vi "Find Top Level.vi"(8 "error in (no error)":errorcluster, 10 "VI":string) -> (0 "error out":errorcluster, 1 "Found?":bool, 2 "Top Level Panel":string)   [LabVIEW 2017, in "MGI-Panel Manager.lvlib" / "Panel Registry.lvclass"]
doc: "Finds the top level panel associated with the VI.\n\n----\nPlease see the following web address for additional documentation and tutorial information:\nhttp://www.mooregoodideas.com/mgi-panel-manager/\n\nAuthor: Derek Trepanier\n\nCopyright (c) 2018, Moore Good Ideas, Inc.\n\nAll rights reserved.\n\nRedistribution and use in source and binary forms, with or without modification, are permitted provided that the following conditions are met:\n\n * Redistributions of source code must retain the above copyright notice, this list of conditions and the following disclaimer.\n * Redistributions in binary form must reproduce the above copyright notice, this list of conditions and the following disclaimer in the documentation and/or other materials provided with the distribution.\n * Neither the name of Moore Good Ideas, Inc. nor the names of its contributors may be used to endorse or promote products derived from this software without specific prior written permission.\n\nTHIS SOFTWARE IS PROVIDED BY THE COPYRIGHT HOLDERS AND CONTRIBUTORS \"AS IS\" AND ANY EXPRESS OR IMPLIED WARRANTIES, INCLUDING, BUT NOT LIMITED TO, THE IMPLIED WARRANTIES OF MERCHANTABILITY AND FITNESS FOR A PARTICULAR PURPOSE ARE DISCLAIMED. IN NO EVENT SHALL THE COPYRIGHT OWNER OR CONTRIBUTORS BE LIABLE FOR ANY DIRECT, INDIRECT, INCIDENTAL, SPECIAL, EXEMPLARY, OR CONSEQUENTIAL DAMAGES (INCLUDING, BUT NOT LIMITED TO, PROCUREMENT OF SUBSTITUTE GOODS OR SERVICES; LOSS OF USE, DATA, OR PROFITS; OR BUSINESS INTERRUPTION) HOWEVER CAUSED AND ON ANY THEORY OF LIABILITY, WHETHER IN CONTRACT, STRICT LIABILITY, OR TORT (INCLUDING NEGLIGENCE OR OTHERWISE) ARISING IN ANY WAY OUT OF THE USE OF THIS SOFTWARE, EVEN IF ADVISED OF THE POSSIBILITY OF SUCH DAMAGE."
uses:
  Panel Registry.lvclass
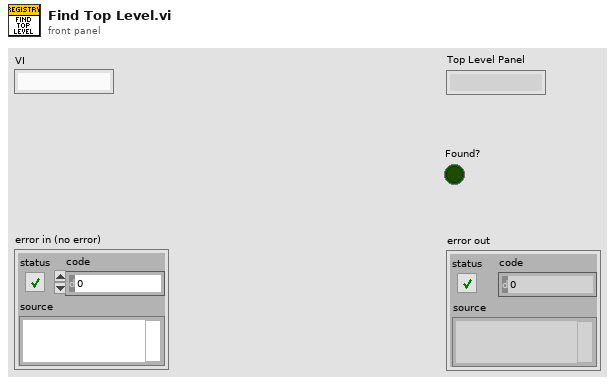
[diagram p1: front panel]
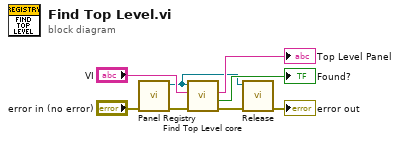
[diagram p0: block diagram]
diagram:
  n1 = call "Panel Registry.vi"("error in (no error)"="error in (no error)") -> ("error out"=w4:errorcluster, "Panel Registry out"=w5:refnum<class "Panel Registry.lvclass">)  [unwired: 9 in]
  n2 = call "Find Top Level core.vi"("error in (no error)"=w4, "VI"="VI", "Panel Registry in"=w5) -> ("error out"=w3:errorcluster, "Found?"=→"Found?":bool, "Top Level Panel"=→"Top Level Panel":string)  [unwired: 6 in]
  n3 = call "Release.vi"("error in (no error)"=w3, "Panel Registry in"=w5) -> ("error out"=→"error out":errorcluster)  [unwired: 9 in]
